vi "Collect Suite Result.vi"(8 "error in (no error)":errorcluster, 10 "Test Suite Result":T1, 11 "Report Generator In":refnum<class "Result Collector.lvclass">) -> (0 "error out":errorcluster, 3 "Report Generator Out":refnum<class "Result Collector.lvclass">)   [LabVIEW 2020, in "Result Collector.lvclass"]
uses:
  Result Collector.lvclass
  Result Types/Suite Results/Test Suite Result.ctl
  Result Types/Assertion Result/Public/TypeDefs/Status.ctl
  Result Types/Case Result/Test Case Result.ctl
  Result Types/Method Result/Method Result.ctl
  Result Types/Assertion Result/Assertion Result.ctl
  Result Types/Assertion Result/Public/TypeDefs/Assertion Type.ctl
  Result Collector.lvclass/Result Collector.ctl
  Result Types/Assertion Result/Assertion Result.lvlib
  Result Types/Method Result/Method Result.lvlib
  Result Types/Case Result/Test Case Result.lvlib
  Result Types/Suite Results/Test Suite Result.lvlib
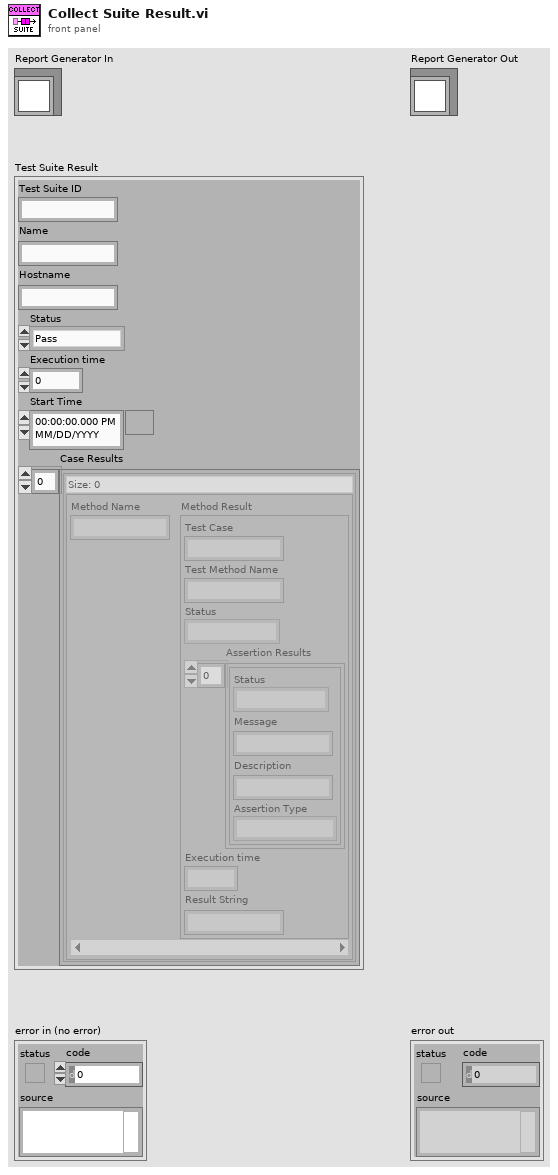
[diagram p1: front panel]
types:
  T1 = typedef "Test Suite Result.lvlib/Test Suite Result.ctl" = cluster{"Test Suite ID":string, "Name":string, "Hostname":string, "Status":T2, "Execution time":dbl, "Start Time":timestamp, "Case Results":T3[]}
  T2 = typedef "Assertion Result.lvlib/Status.ctl" = enum16{"Pass", "Fail", "Error", "Skipped", "Setup Error", "Broken", "Teardown Error"}
  T3 = typedef "Test Case Result.lvlib/Test Case Result.ctl" = map{string, T4}
  T4 = typedef "Method Result.lvlib/Method Result.ctl" = cluster{"Test Case":string, "Test Method Name":string, "Status":T2, "Assertion Results":T5[], "Execution time":dbl, "Result String":string}
  T5 = typedef "Assertion Result.lvlib/Assertion Result.ctl" = cluster{"Status":T2, "Message":string, "Description":string, "Assertion Type":T6}
  T6 = typedef "Assertion Result.lvlib/Assertion Type.ctl" = enum16{"None", "Pass", "Fail", "Skip", "Pass if Equal", "Fail if Equal", "Pass if Error", "Fail if Error", "Pass if", "Fail if"}
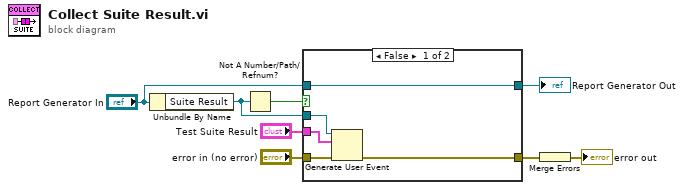
[diagram p0: block diagram]
diagram:
  n1 = Unbundle By Name("Report Generator In") -> ("Suite Result"=w7:refnum<user-event>)
  n2 = Not A Number/Path/Refnum?(number/path/refnum=w7) -> (NaN/Path/Refnum?=w8:bool)
  n3 = case shown="False" w8 {
    tunnel: "Test Suite Result" -> [w9 _]
    tunnel: "error in (no error)" -> [w13 w15]
    tunnel: [w12 w15] -> w6
    tunnel: w7 -> [w11 _]
    tunnel: "Report Generator In" -> [w10 w14]
    tunnel: [w10 w14] -> w1
    frame False {
      n4 = Generate User Event(user event=w11, event data cluster=w9, error in=w13) -> (error out=w12:errorcluster)  [unwired: 1 in, 1 out]
    }
    frame True {
      # "Report generator not initialized,\ndiscard results."
    }
  }
  "Report Generator Out" <- w1
  n5 = Merge Errors(w6) -> (→"error out":errorcluster)
